vi "计算结果-步响应-缩入实测.vi"(3 "步响应计算参数 in":T1, 4 "步响应控制参数":T2={"rise_step"=1.0, "rise_criterion"=600.0, "peak_step"=1.0, "peak_criterion"=50.0, "nb_of_peaks"=200.0}, 5 "行程 in":dbl[](array[numeric])) -> (0 "步响应计算参数 out":T1, 2 "行程 out":dbl[](array[numeric]))   [LabVIEW 2013]
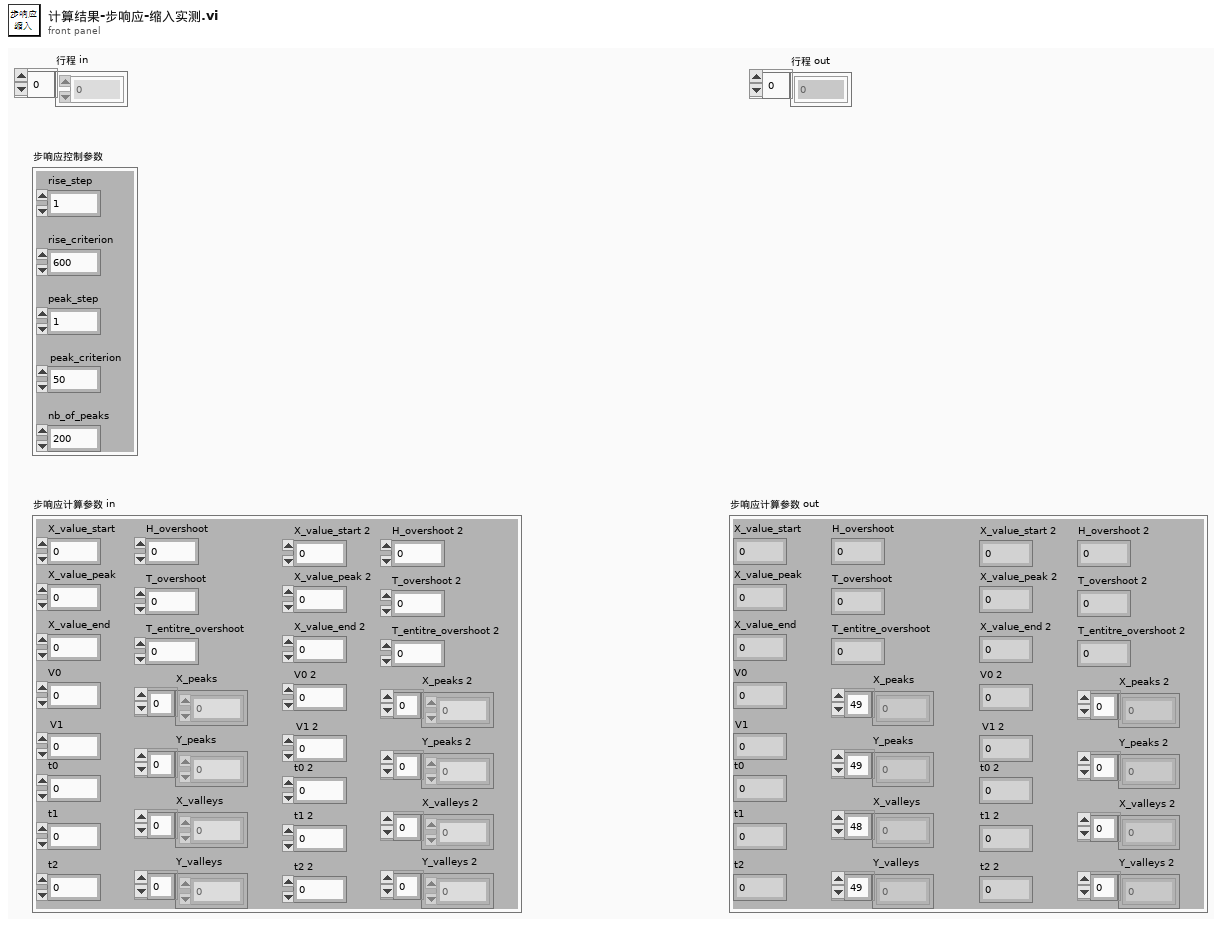
[diagram p1: front panel]
types:
  T1 = cluster{"X_value_start":dbl, "X_value_peak":dbl, "t1":dbl, "X_value_end":dbl, "V0":dbl, "V1":dbl, "t0":dbl, "X_peaks":dbl[], "X_valleys":dbl[], "Y_peaks":dbl[], "Y_valleys":dbl[], "t2":dbl, "H_overshoot":dbl, "T_overshoot":dbl, "T_entitre_overshoot":dbl, "X_value_start 2":dbl, "X_value_peak 2":dbl, "t1 2":dbl, "X_value_end 2":dbl, "V0 2":dbl, "V1 2":dbl, "t0 2":dbl, "X_peaks 2":dbl[], "X_valleys 2":dbl[], "Y_peaks 2":dbl[], "t2 2":dbl, "H_overshoot 2":dbl, "T_overshoot 2":dbl, "T_entitre_overshoot 2":dbl, "Y_valleys 2":dbl[]}
  T2 = cluster{"rise_step":dbl, "rise_criterion":dbl, "peak_step":dbl, "peak_criterion":dbl, "nb_of_peaks":dbl}
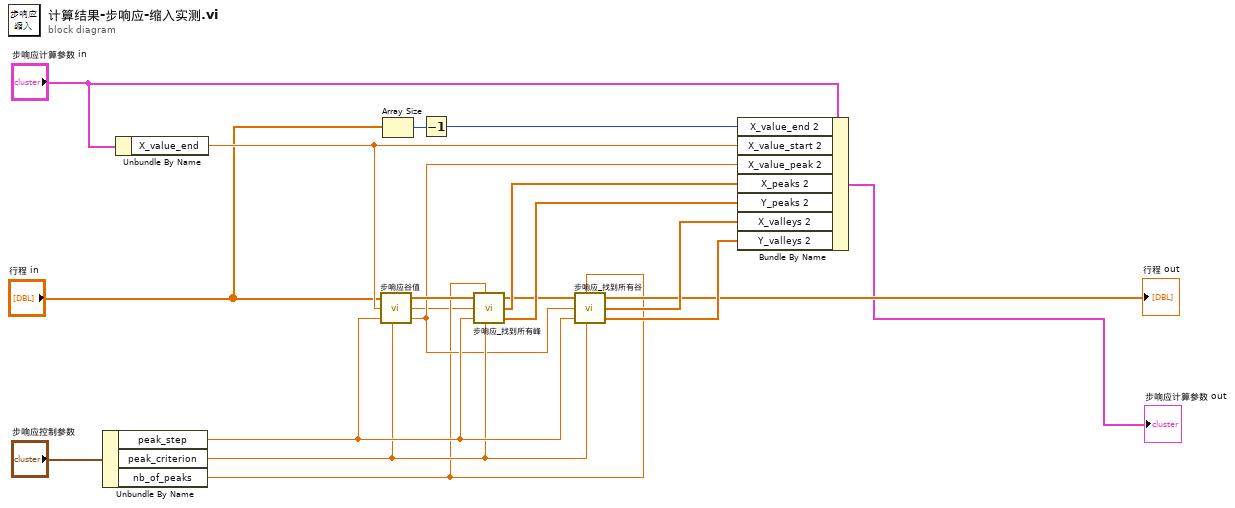
[diagram p0: block diagram]
diagram:
  n1 = Unbundle By Name("步响应控制参数") -> ("peak_step"=w17:dbl, "peak_criterion"=w16:dbl, "nb_of_peaks"=w9:dbl)
  n2 = Unbundle By Name("步响应计算参数 in") -> ("X_value_end"=w7:dbl)
  n3 = call "步响应谷值.vi"("行程 in"="行程 in", "X_start"=w7, "step_valley"=w17, "（要求）连续大于0的次数"=w16) -> ("行程 out"=w19:dbl[], "X_value"=w5:dbl, "X_value_next"=w11:dbl)  [unwired: 1 in]
  n4 = Array Size(array="行程 in") -> (size(s)=w4:i32)
  n5 = Decrement(x=w4) -> (x-1=w3:i32)
  n6 = call "步响应_找到所有峰.vi"("行程 in"=w19, "nb_of_peaks"=w9, "X_peak_start"=w5, "step_peak"=w17, "（要求）连续大于0的次数"=w16) -> ("行程 out"=w6:dbl[], "X_Peaks"=w13:dbl[], "Y_Peaks"=w12:dbl[])
  n7 = call "步响应_找到所有谷.vi"("行程 in"=w6, "nb_of_peaks"=w9, "X_valley_start"=w11, "step_valley"=w17, "（要求）连续大于0的次数"=w16) -> ("行程 out"=→"行程 out":dbl[], "X_valley"=w15:dbl[], "Y_valley"=w14:dbl[])
  n8 = Bundle By Name(cluster="步响应计算参数 in", "X_value_end 2"=w3, "X_value_start 2"=w7, "X_value_peak 2"=w11, "X_peaks 2"=w13, "Y_peaks 2"=w12, "X_valleys 2"=w15, "Y_valleys 2"=w14) -> (→"步响应计算参数 out":T1)
